vi "gun_fir_averaging.vi"(11 "Raw":dbl) -> (3 "Filt":dbl)   [LabVIEW 2011]
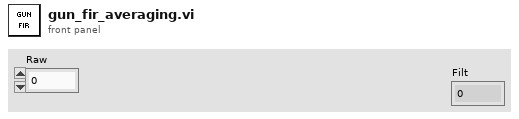
[diagram p1: front panel]
types:
  T1 = cluster{"Raw":dbl, "Raw":dbl, "Raw":dbl, "Raw":dbl}
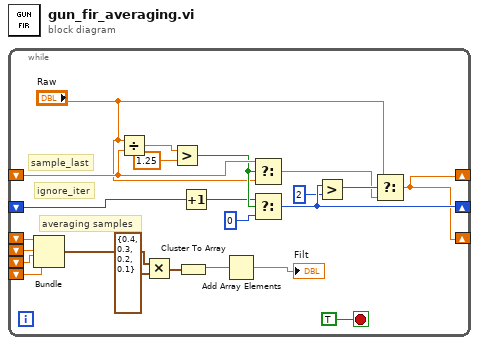
[diagram p0: block diagram]
diagram:
  n1 = while {
    shift-right: [w11] -> _
    shift-left: _ -> [w20]
    shift-right: [w11] -> _
    shift-left: _ -> [w10]
    shift-right: [w15] -> _
    shift-left: _ -> [w17]
    shift-left: _ -> [w9]
    shift-left: _ -> [w8]
    shift-left: _ -> [w7]
    stop <- TRUE stop-if-true
    # "averaging samples"
    # "ignore_iter"
    # "sample_last"
    n2 = Bundle("Raw"=w10, "Raw"=w9, "Raw"=w8, "Raw"=w7) -> (w6:T1)  [unwired: 1 in]
    n3 = Divide(x="Raw", y=w20) -> (x/y=w22:dbl)
    n4 = Multiply(x=w6, y=T1 {"Raw"=0.4, "Raw"=0.3, "Raw"=0.2, "Raw"=0.1}) -> (x*y=w4:T1)
    n5 = Greater?(x=w22, y=1.25) -> (0:w19:bool)
    n6 = Cluster To Array(cluster=w4) -> (array=w3:dbl[])
    n7 = Increment(x=w17) -> (x+1=w18:i32)
    n8 = Add Array Elements(numeric array=w3) -> (sum=→"Filt":dbl)
    n9 = Select(t=w20, s=w19, f="Raw") -> (s? t:f=w12:dbl)
    n10 = Select(t=w18, s=w19, f=0) -> (s? t:f=w15:i32)
    n11 = Greater?(x=w15, y=2) -> (0:w13:bool)
    n12 = Select(t="Raw", s=w13, f=w12) -> (s? t:f=w11:dbl)
  }
